vi "Round (SubVI).vi"(11 "Numeric in":dbl) -> (3 "Numeric out":dbl)   [LabVIEW 2021]
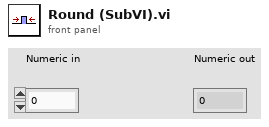
[diagram p1: front panel]
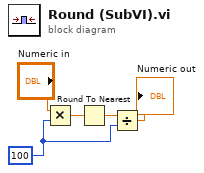
[diagram p0: block diagram]
diagram:
  w4 = 100
  n1 = Multiply(x="Numeric in", y=w4) -> (x*y=w2:dbl)
  n2 = Round To Nearest(number=w2) -> (nearest integer value=w3:dbl)
  n3 = Divide(x=w3, y=w4) -> (x/y=→"Numeric out":dbl)
